vi "Find LPC.vi"(8 "error in (no error)":errorcluster, 11 "VISA resource name":refnum<visa-resource-name>="GPIB0::8::INSTR") -> (0 "error out":errorcluster, 2 "LPC found?":bool, 3 "VISA resource name out":refnum<visa-resource-name>)   [LabVIEW 2012, in "BEOC LPC.lvlib"]
doc: "Checks for the LPC (laser power controller, aka power stabilizer)."
uses:
  BEOC LPC.lvlib
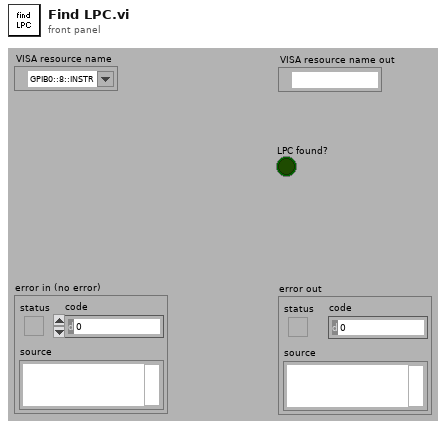
[diagram p1: front panel]
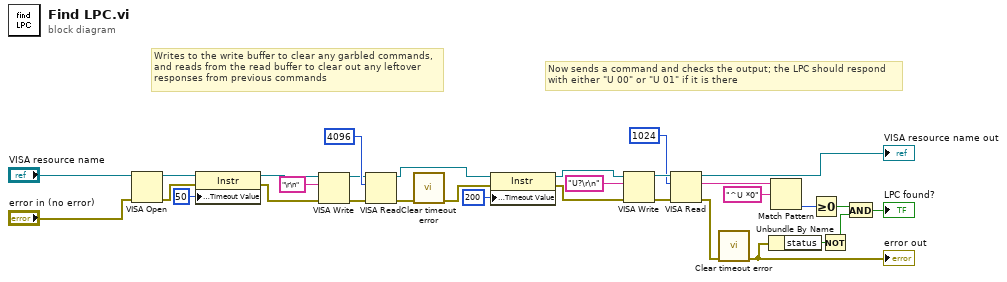
[diagram p0: block diagram]
diagram:
  # "Now sends a command and checks the output; the LPC should respond with either \"U 00\" or \"U 01\" if it is there"
  # "Writes to the write buffer to clear any garbled commands, and reads from the read buffer to clear out any leftover responses from previous commands"
  n1 = VISA Open(error in (no error)="error in (no error)", VISA resource name="VISA resource name") -> (VISA resource name=w29:refnum<visa-resource-name>, error out=w28:errorcluster)  [unwired: 3 out]
  n2 = property class="Instr"(reference=w29, error in=w28, "General Settings:Timeout Value"=u32 50) -> (reference out=w8:refnum<visa-resource-name>, error out=w6:errorcluster)
  n3 = VISA Write(VISA resource name=w8, write buffer="\r\n" ("write string"), error in (no error)=w6) -> (VISA resource name out=w7:refnum<visa-resource-name>, error out=w5:errorcluster)  [unwired: 1 out]
  n4 = VISA Read(VISA resource name=w7, byte count=u32 4096, error in (no error)=w5) -> (VISA resource name out=w16:refnum<visa-resource-name>, error out=w19:errorcluster)  [unwired: 2 out]
  n5 = call "Clear timeout error.vi"("error in (no error)"=w19) -> ("error out"=w17:errorcluster)  [unwired: 1 in, 9 out]
  n6 = property class="Instr"(reference=w16, error in=w17, "General Settings:Timeout Value"=u32 200) -> (reference out=w15:refnum<visa-resource-name>, error out=w14:errorcluster)
  n7 = VISA Write(VISA resource name=w15, write buffer="U?\r\n" ("write string"), error in (no error)=w14) -> (VISA resource name out=w24:refnum<visa-resource-name>, error out=w25:errorcluster)  [unwired: 1 out]
  n8 = VISA Read(VISA resource name=w24, byte count=u32 1024, error in (no error)=w25) -> (VISA resource name out=→"VISA resource name out":refnum<visa-resource-name>, read buffer=w13:string, error out=w26:errorcluster)  [unwired: 1 out]
  n9 = call "Clear timeout error.vi"("error in (no error)"=w26) -> ("error out"=w10:errorcluster)  [unwired: 1 in, 9 out]
  "error out" <- w10
  n10 = Unbundle By Name(w10) -> ("status"=w4:bool)
  n11 = Match Pattern(string=w13, regular expression="^U *0") -> (offset past match=w11:i32)  [unwired: 4 out]
  n12 = Greater Or Equal To 0?(x=w11) -> (x >= 0?=w3:bool)
  n13 = Not(x=w4) -> (.not. x?=w2:bool)
  n14 = And(x=w3, y=w2) -> (x .and. y?=→"LPC found?":bool)
